vi "module-04-and-nand.vi"() -> ()   [LabVIEW 2019]
panel:
  in  "?":enum32{"Execution", "Logic"}(tab)
  out "Digital State Chart":T1(graph)
  in  "Input":bool
  in  "Input 2":bool
  in  "Input 3":bool
  in  "Input 4":bool
  in  "Not Input 5":bool
  in  "Not Input 6":bool
  in  "Not Input 7":bool
  in  "Not Input 8":bool
  out "Ouptut":bool
  in  "Cycle \nMilliseconds":u32=100 min=10 max=30000 step=10
  # "AND NAND GATE TEST\nInputs 1-4 AND\nInputs 5-8 NOT - AND"
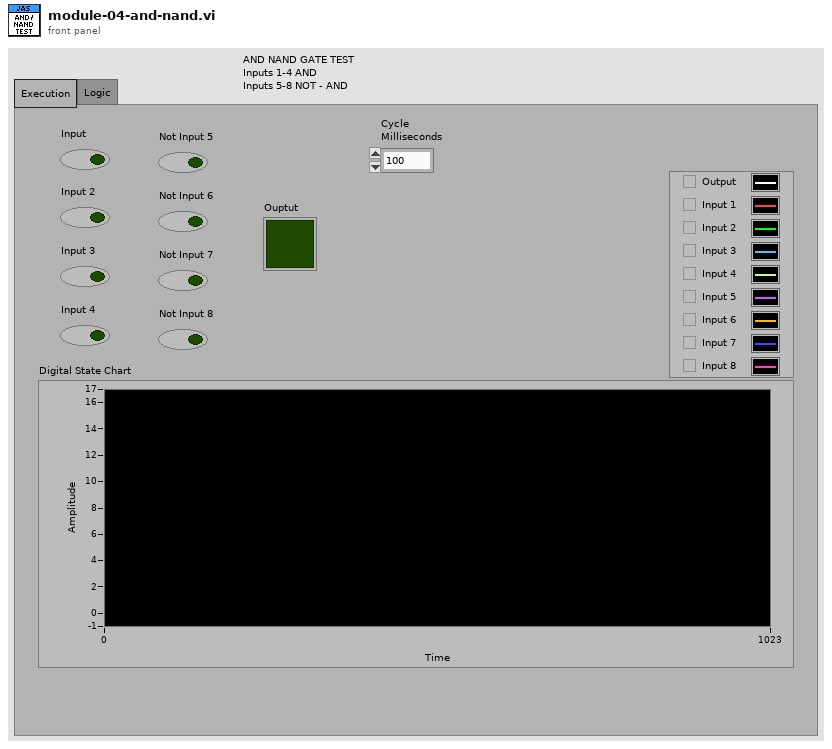
[diagram p1: front panel]
types:
  T1 = cluster{dbl, dbl, dbl, dbl, dbl, dbl, dbl, dbl, dbl}
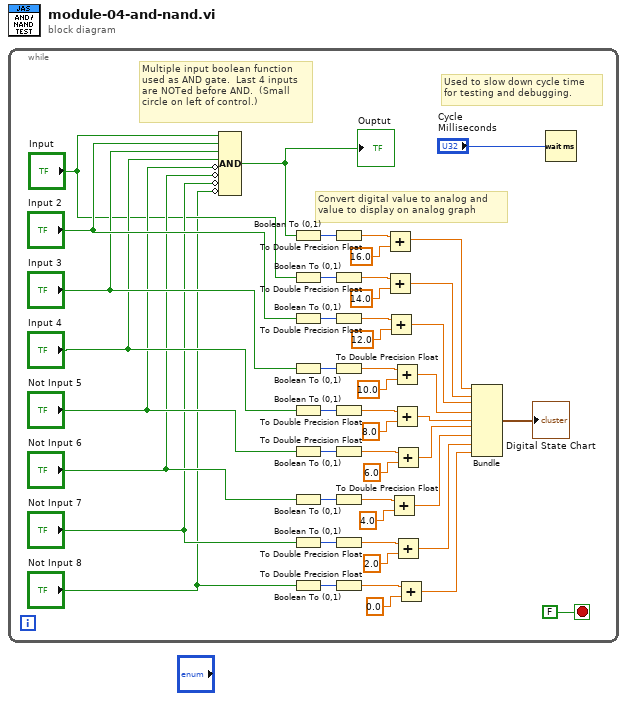
[diagram p0: block diagram]
diagram:
  n1 = while {
    stop <- FALSE stop-if-true
    # "Used to slow down cycle time\nfor testing and debugging."
    # "Multiple input boolean function\nused as AND gate.  Last 4 inputs\nare NOTed before AND.  (Small\ncircle on left of control.)"
    # "Convert digital value to analog and \nvalue to display on analog graph"
    n2 = Compound Arithmetic op=AND("Input", "Input 2", "Input 3", "Input 4", invert "Not Input 5", invert "Not Input 6", invert "Not Input 7", invert "Not Input 8") -> (w9:bool)
    "Ouptut" <- w9
    n3 = Boolean To (0,1)(Boolean=w9) -> (0, 1=w24:i16)
    n4 = Boolean To (0,1)(Boolean="Input") -> (0, 1=w25:i16)
    n5 = Boolean To (0,1)(Boolean="Input 2") -> (0, 1=w27:i16)
    n6 = Boolean To (0,1)(Boolean="Input 3") -> (0, 1=w36:i16)
    n7 = Boolean To (0,1)(Boolean="Input 4") -> (0, 1=w39:i16)
    n8 = Boolean To (0,1)(Boolean="Not Input 5") -> (0, 1=w41:i16)
    n9 = Boolean To (0,1)(Boolean="Not Input 6") -> (0, 1=w37:i16)
    n10 = Boolean To (0,1)(Boolean="Not Input 7") -> (0, 1=w43:i16)
    n11 = Boolean To (0,1)(Boolean="Not Input 8") -> (0, 1=w45:i16)
    n12 = To Double Precision Float(number=w24) -> (double precision float=w29:dbl)
    n13 = To Double Precision Float(number=w25) -> (double precision float=w26:dbl)
    n14 = To Double Precision Float(number=w27) -> (double precision float=w28:dbl)
    n15 = To Double Precision Float(number=w36) -> (double precision float=w47:dbl)
    n16 = To Double Precision Float(number=w39) -> (double precision float=w40:dbl)
    n17 = To Double Precision Float(number=w41) -> (double precision float=w42:dbl)
    n18 = To Double Precision Float(number=w37) -> (double precision float=w38:dbl)
    n19 = To Double Precision Float(number=w43) -> (double precision float=w44:dbl)
    n20 = To Double Precision Float(number=w45) -> (double precision float=w46:dbl)
    n21 = Add(x=w29, y=16.0) -> (x+y=w20:dbl)
    n22 = Add(x=w26, y=14.0) -> (x+y=w19:dbl)
    n23 = Add(x=w28, y=12.0) -> (x+y=w18:dbl)
    n24 = Add(x=w38, y=4.0) -> (x+y=w11:dbl)
    n25 = Add(x=w47, y=10.0) -> (x+y=w17:dbl)
    n26 = Add(x=w40, y=8.0) -> (x+y=w16:dbl)
    n27 = Add(x=w42, y=6.0) -> (x+y=w15:dbl)
    n28 = Add(x=w44, y=2.0) -> (x+y=w14:dbl)
    n29 = Add(x=w46, y=0.0) -> (x+y=w13:dbl)
    n30 = Bundle(w20, w19, w18, w17, w16, w15, w11, w14, w13) -> (→"Digital State Chart":T1)  [unwired: 1 in]
    n31 = Wait (ms)(milliseconds to wait="Cycle \nMilliseconds") -> ()  [unwired: 1 out]
  }
